vi "Find_Number_LineMARVIN.vi"(4 "Test Paragraph":string, 5 "error in":errorcluster, 8 "Row Headers[]":string[](array[string])) -> (0 "error out":errorcluster, 1 "1 line Test ?":bool, 2 "Found":bool, 3 "Line number":i32)   [LabVIEW 2017]
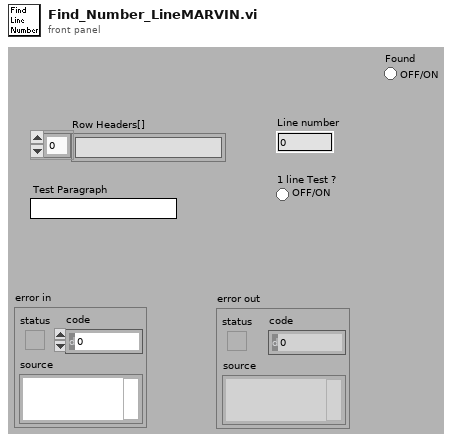
[diagram p1: front panel]
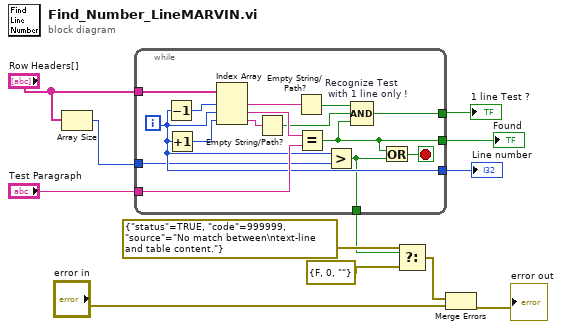
[diagram p0: block diagram]
diagram:
  n1 = Array Size(array="Row Headers[]") -> (size(s)=w8:i32)
  n2 = while {
    tunnel: "Test Paragraph" -> [w27]
    tunnel: "Row Headers[]" -> [w26]
    tunnel: [w17] -> w11
    tunnel: [w16] -> w12
    tunnel: w8 -> [w15]
    tunnel: [w14] -> w4
    tunnel: [w13] -> w1
    i -> [w16]
    stop <- w18 stop-if-true
    n3 = Decrement(x=w16) -> (x-1=w25:i32)
    n4 = Increment(x=w16) -> (x+1=w24:i32)
    n5 = Index Array(array=w26, index #1=w25, index #2=w16, index #3=w24) -> (element #1=w22:string, element #2=w23:string, element #3=w21:string)
    n6 = Empty String/Path?(string/path=w21) -> (empty?=w19:bool)
    n7 = Empty String/Path?(string/path=w22) -> (empty?=w20:bool)
    n8 = Equal?(x=w23, y=w27) -> (x = y?=w13:bool)
    n9 = Greater?(x=w16, y=w15) -> (0:w14:bool)
    n10 = Compound Arithmetic op=AND "Recognize Test \n with 1 line only !"(w20, w19, w13) -> (w17:bool)
    n11 = Or(x=w13, y=w14) -> (x .or. y?=w18:bool)
  }
  "Line number" <- w12
  "1 line Test ?" <- w11
  "Found" <- w1
  n12 = Select(t=errorcluster {"status"=TRUE, "code"=999999, "source"="No match between\ntext-line and table content."} ("error in 1 (no error)"), s=w4, f=errorcluster {"status"=FALSE, "code"=0, "source"=""}) -> (s? t:f=w2:errorcluster)
  n13 = Merge Errors(w2, "error in") -> (→"error out":errorcluster)
